vi "NI VeriStand - Close Custom Device Reference.vi"(8 "error in (no error)":errorcluster, 11 "Custom Device":T1) -> (0 "error out":errorcluster)   [LabVIEW 2020, in "NI_VS Custom Device ExecutionAPI.lvlib"]
doc: "Closes an open reference to a custom device. This VI acts on references you open to send messages to a custom device, such as references the Open Custom Device Reference creates."
uses:
  <vilib>/NI VeriStand/Execution/CustomDevice/NI_VS Custom Device ExecutionAPI.lvlib
  <vilib>/NI VeriStand/Execution/CustomDevice/Custom Device Ref.ctl
  NationalInstruments.VeriStand.ClientAPI
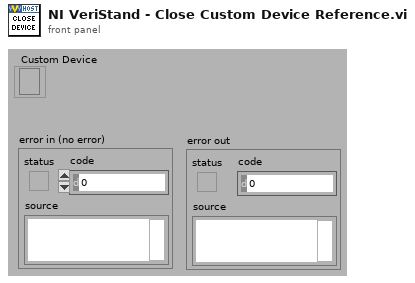
[diagram p1: front panel]
types:
  T1 = typedef "NI_VS Custom Device ExecutionAPI.lvlib/Custom Device Ref.ctl" = refnum<k24>
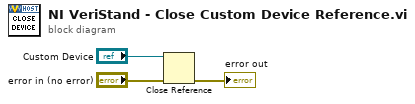
[diagram p0: block diagram]
diagram:
  n1 = Close Reference(reference="Custom Device", error in (no error)="error in (no error)") -> (error out=→"error out":errorcluster)
